vi "Param init.vi"(8 "error in (no error)":errorcluster, 10 "N_param":i32) -> (0 "error":errorcluster, 3 "Param":T1)   [LabVIEW 2019, in "Inputs.lvlib"]
uses:
  Inputs.lvlib
  Ctl/Param.ctl
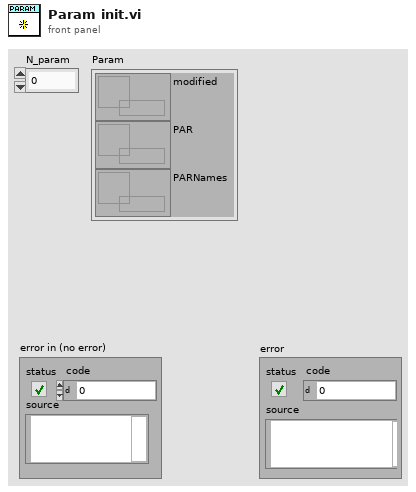
[diagram p1: front panel]
types:
  T1 = typedef "Inputs.lvlib/Param.ctl" = cluster{"modified":refnum<data-value>, "PAR":refnum<data-value>, "PARNames":refnum<data-value>}
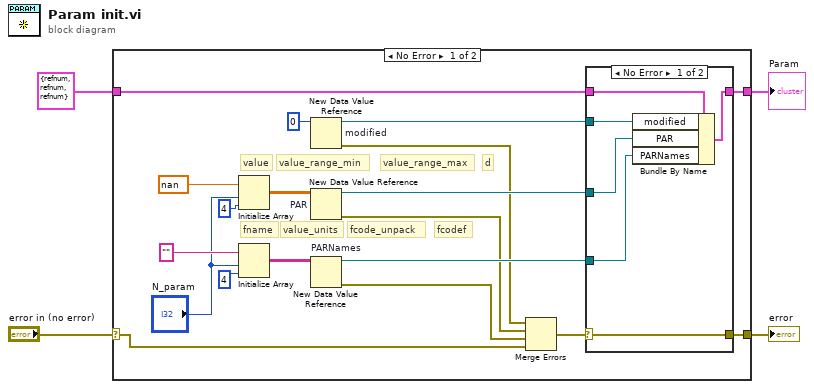
[diagram p0: block diagram]
diagram:
  n1 = case shown="No Error" "error in (no error)" {
    selector: "error in (no error)" -> [w11 w33]
    tunnel: [w23 w33] -> w4
    tunnel: [w22 w32] -> w3
    tunnel: T1 {"modified"=refnum, "PAR"=refnum, "PARNames"=refnum} ("Param") -> [w12 w32]
    frame No Error {
      # "fcodef"
      # "fcode_unpack"
      # "value_units"
      # "fname"
      # "d"
      # "value_range_max"
      # "value_range_min"
      # "value"
      n2 = Initialize Array(nan ("PAR"), "N_param", 4 ("dimension size")) -> (w10:dbl[][])
      n3 = Initialize Array("" ("PARNames"), "N_param", 4 ("dimension size")) -> (w17:string[][])
      n4 = New Data Value Reference "modified"(data value=u8 0 ("modified")) -> (data value reference=w7:refnum<data-value>, error out=w6:errorcluster)  [unwired: 1 in]
      n5 = New Data Value Reference "PAR"(data value=w10) -> (data value reference=w9:refnum<data-value>, error out=w8:errorcluster)  [unwired: 1 in]
      n6 = New Data Value Reference "PARNames"(data value=w17) -> (data value reference=w15:refnum<data-value>, error out=w16:errorcluster)  [unwired: 1 in]
      n7 = Merge Errors(w6, w8, w16, w11) -> (w14:errorcluster)
      n8 = case shown="No Error" w14 {
        selector: w14 -> [w27 w31]
        tunnel: w9 -> [w25 _]
        tunnel: [w27 w31] -> w23
        tunnel: w12 -> [w29 w30]
        tunnel: [w28 w30] -> w22
        tunnel: w15 -> [w26 _]
        tunnel: w7 -> [w24 _]
        frame No Error {
          n9 = Bundle By Name(cluster=w29, "modified"=w24, "PAR"=w25, "PARNames"=w26) -> (w28:T1)
        }
        frame Error {
        }
      }
    }
    frame Error {
    }
  }
  "error" <- w4
  "Param" <- w3
